vi "Initialize-errors.vi"(8 "error in (no error)":errorcluster, 11 "Data ref. in":refnum<data-value>) -> (0 "error out":errorcluster, 3 "Data ref.":refnum<data-value>)   [LabVIEW 2013, in "CameraVision.lvlib" / "CV-Main.lvclass"]
uses:
  CV-Main.lvclass
  Errors/Settings.ctl
  Errors/Languages.ctl
  CV-Main.lvclass/CV-Main.ctl
  Storage/CV-Storage.lvclass/CV-Storage.ctl
  Storage/Read Base path.vi
  Errors/CV-Errors.lvclass
  Storage/CV-Storage.lvclass
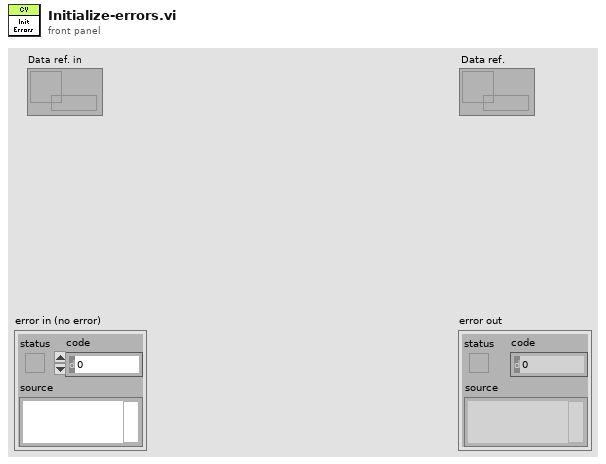
[diagram p1: front panel]
types:
  T1 = typedef "CameraVision.lvlib/CV-Errors.lvclass/Settings.ctl" = cluster{"Language":T2, "Display error dialog":bool, "Write log to file":bool, "Stream to log file":bool, "Overwrite existing log":bool, "Max log size":i32, "Max number of log files":i32}
  T2 = typedef "CameraVision.lvlib/CV-Errors.lvclass/Languages.ctl" = enum16{"English"}
  T3 = typedef "CameraVision.lvlib/CV-Errors.lvclass/Object-reference.ctl" = refnum<data-value>
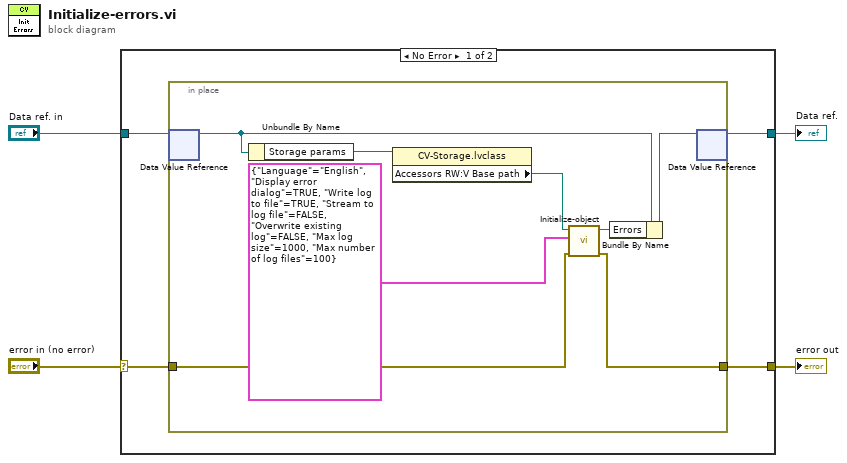
[diagram p0: block diagram]
diagram:
  n1 = case shown="No Error" "error in (no error)" {
    selector: "error in (no error)" -> [w6 w18]
    tunnel: [w5 w18] -> w3
    tunnel: "Data ref. in" -> [w8 w17]
    tunnel: [w7 w17] -> w1
    frame No Error {
      n2 = in-place {
        in-place-border: [w13] -> w5
        in-place-border: w6 -> [w14]
        n3 = in-place-dvr #1(w8) -> (w11:refnum<class "CV-Main.lvclass">)  [unwired: 1 out]
        n4 = Unbundle By Name(w11) -> ("Storage params"=w10:refnum<data-value>)
        n5 = property class="CV-Storage.lvclass"(reference=w10) -> ("Accessors RW:V Base path"=w9:path)  [unwired: 1 in, 2 out]
        n6 = call "Initialize-object.vi"("error in (no error)"=w14, "Settings"=T1 {"Language"=enum."English", "Display error dialog"=TRUE, "Write log to file"=TRUE, "Stream to log file"=FALSE, "Overwrite existing log"=FALSE, "Max log size"=1000, "Max number of log files"=100}, "Base path"=w9) -> ("error out"=w13:errorcluster, "Errors out"=w15:T3)  [unwired: 7 in]
        n7 = Bundle By Name(cluster=w11, "Errors"=w15) -> (w16:refnum<class "CV-Main.lvclass">)
        n8 = in-place-dvr #1(w16) -> (w7:refnum<data-value>)  [unwired: 1 out]
      }
    }
    frame Error {
    }
  }
  "error out" <- w3
  "Data ref." <- w1
